vi "PCert-ConfigPageNF-Tell.vi"(8 "error in (no error)":errorcluster, 9 "Message Body":string, 10 "Message Header":string="Testing", 11 "ERP-ConfigPageNF in":refnum<class "PCert-ConfigPageNF.lvclass">) -> (0 "error out":errorcluster, 3 "ERP-ConfigPageNF out":refnum<class "PCert-ConfigPageNF.lvclass">)   [LabVIEW 2013, in "PCert-ConfigPageNF.lvclass"]
uses:
  PCert-ConfigPageNF.lvclass
  PCert-ConfigPageNF.lvclass/PCert-ConfigPageNF.ctl
  ftw-dataflow/Actor/src/Connector/FTW-ActorConnector.lvclass
panel:
  out "Timed out?":bool
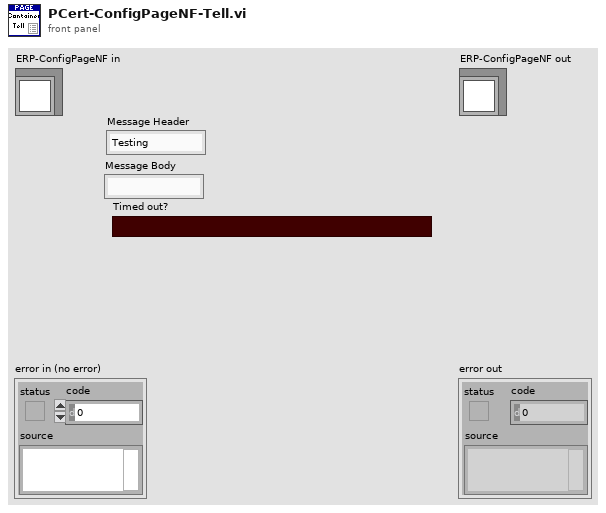
[diagram p1: front panel]
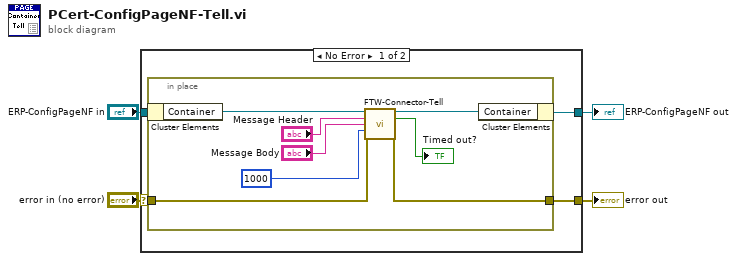
[diagram p0: block diagram]
diagram:
  n1 = case shown="No Error" "error in (no error)" {
    selector: "error in (no error)" -> [w8 w18]
    tunnel: [w7 w18] -> w3
    tunnel: [w5 w17] -> w1
    tunnel: "ERP-ConfigPageNF in" -> [w6 w17]
    frame No Error {
      n2 = in-place {
        in-place-border: w8 -> [w12]
        in-place-border: [w11] -> w7
        n3 = in-place-cluster #1(w6) -> ("Container"=w16:refnum<class "FTW-ActorConnector.lvclass">)
        n4 = call "FTW-Connector-Tell.vi"("FTW Actor Connector"=w16, "Message Header"="Message Header", "Message Body"="Message Body", "Timeout"=1000, "error in"=w12) -> ("FTW Actor Connector out"=w15:refnum<class "FTW-ActorConnector.lvclass">, "Timed out?"=→"Timed out?":bool, "error out"=w11:errorcluster)  [unwired: 8 in]
        n5 = in-place-cluster #1("Container"=w15) -> (w5:refnum<class "PCert-ConfigPageNF.lvclass">)
      }
    }
    frame Error {
    }
  }
  "error out" <- w3
  "ERP-ConfigPageNF out" <- w1
